vi "Channel 1.vi"() -> ()   [LabVIEW 2016]
panel:
  in  "Channel Name 1":string="Channel 1"
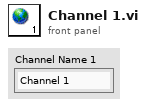
[diagram p1: front panel]
diagram:
